vi "Connect to Target.vi"(8 "error in (no error)":errorcluster, 11 "SV B-M (Host) in":refnum<class "SV B-M (Host).lvclass">) -> (0 "error out":errorcluster, 3 "SV B-M (Host) out":refnum<class "SV B-M (Host).lvclass">)   [LabVIEW 2015, in "SV B-M (Host).lvclass"]
doc: "Connect to the target by opening command & ack network streams."
uses:
  SV B-M (Host).lvclass
  Listbox - In Progress.vi
  Command & Ack - Create Endpoints.vi
  Listbox - Complete.vi
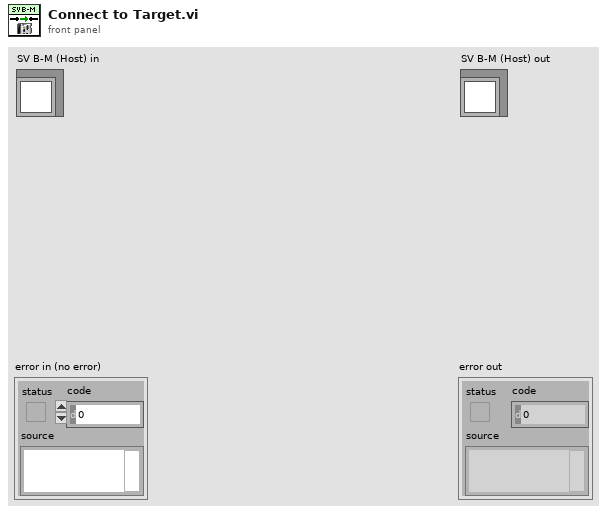
[diagram p1: front panel]
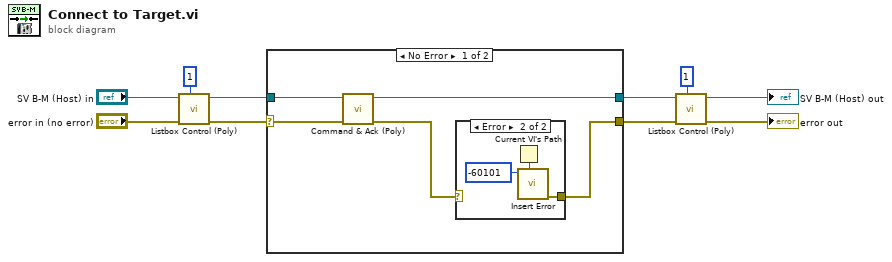
[diagram p0: block diagram]
diagram:
  n1 = call-poly "Listbox Control (Poly).vi"("Row to Update"=1, "error in (no error)"="error in (no error)", "SV B-M In"="SV B-M (Host) in") -> ("error out"=w4:errorcluster, "SV B-M Out"=w5:refnum<class "SV B-M (Host).lvclass">)  [unwired: 7 in]
  n2 = case shown="No Error" w4 {
    selector: w4 -> [w15 w21]
    tunnel: [w11 w21] -> w3
    tunnel: [w13 w20] -> w6
    tunnel: w5 -> [w14 w20]
    frame No Error {
      n3 = call-poly "Command & Ack (Poly).vi"("error in (no error)"=w15, "SV B-M (Host) in"=w14) -> ("error out"=w12:errorcluster, "SV B-M (Host) out"=w13:refnum<class "SV B-M (Host).lvclass">)  [unwired: 8 in]
      n4 = case shown="Error" w12 {
        selector: w12 -> [w16 _]
        tunnel: [w16 w19] -> w11
        frame No Error {
        }
        frame Error {
          n5 = Current VI's Path() -> (path=w17:path)
          n6 = call "Insert Error.vi"("VI Path"=w17, "Error Code"=-60101) -> ("error out"=w19:errorcluster)  [unwired: 9 in]
        }
      }
    }
    frame Error {
    }
  }
  n7 = call-poly "Listbox Control (Poly).vi"("Row to Update"=1, "error in (no error)"=w3, "SV B-M In"=w6) -> ("error out"=→"error out":errorcluster, "SV B-M Out"=→"SV B-M (Host) out":refnum<class "SV B-M (Host).lvclass">)  [unwired: 7 in]
